vi "JSONtoLV-DBUpdate.vi"(8 "error in":errorcluster, 11 "Input JSON Object":string) -> (0 "error out":errorcluster, 3 "value":T1)   [LabVIEW 2013]
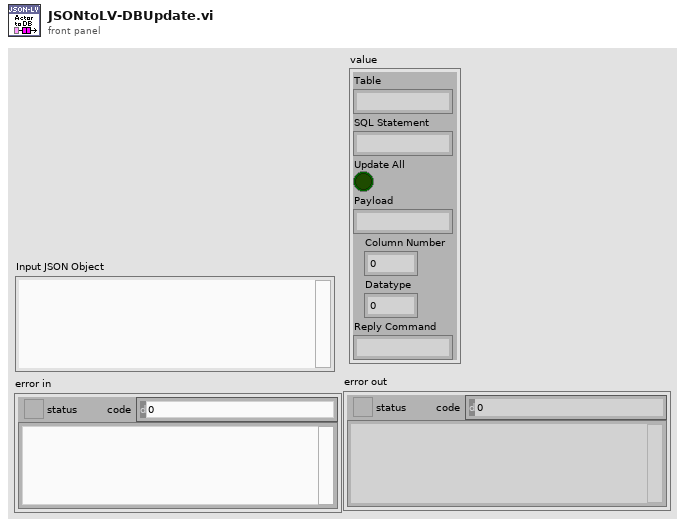
[diagram p1: front panel]
types:
  T1 = cluster{"Table":string, "SQL Statement":string, "Update All":bool, "Payload":string, "Column Number":i32, "Datatype":i32, "Reply Command":string}
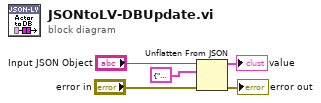
[diagram p0: block diagram]
diagram:
  n1 = Unflatten From JSON(JSON string="Input JSON Object", type and defaults=T1 {"Table"="", "SQL Statement"="", "Update All"=FALSE, "Payload"="", "Column Number"=0, "Datatype"=0, "Reply Command"=""} ("output cluster"), error in (no error)="error in") -> (value=→"value":T1, error out=→"error out":errorcluster)  [unwired: 4 in]
